vi "TSCAN_CAN_Table.vi"(8 "Data输入":T2={"Communication message"={"Sender"="", "receiver"="", "message"="", "data"=variant}, "Data"={"Config_parameter"={"Bus_Type"=0, "Channel"=0, "Channels used"=0, "DLL_PATH"=path "", "Read message type"=1, "REC_Channel"=0}, "Send_parameter"={"SendData"=[], "Data Length"=0, "ID"=0, "Frame Format"=0, "Frame Type"=0, "BRS"=enum."Close", "FD Frame"=0, "async&sync"=enum."async", "Timeout"=0}, "DBC_Ctr"={"DBC Path"=path "", "DBC loading channel"=0, "DatabaseId"=0, "DBMessages"=[], "DBSignals"=[]}, "CAN_Config_Array"=[], "CANFD_Config_Array"=[], "CAN_Config_Regs_Array"=[], "CANFD_Config_Regs_Array"=[], "Blf_Log"={"Blf_Log_PATH"=path ""}, "UDS"={"UDS Control"={"UDS Channel Index"=0, "Request ID"=1992, "Response ID"=2015, "Request ID (Func)"=1, "Session Mode"=1, "Reset Mode"=255, "DTC Mask"=0, "GropOfDTC"=0, "Seed Level"=2, "Seed"=[], "Key Level"=0, "Key"=[], "Read Identifier"=0, "UDS Read Data"=[], "ASCII Data"="", "Write Identifier"=0, "UDS Wrtie Data"=[], "IO Control Identifier"=1, "UDS IOControl Data"=[], "IO Control Mode"=0, "UDS IOControl Read Data"=[], "Routine Control Identifier"=0, "UDS RoutineControl Data"=[], "UDS RoutineControl Read Data"=[], "Routine Control Mode"=1, "SupportFDCAN"=TRUE, "time config"={"p2_timeout"=0, "p2_extended"=0, "s3_servertime"=0, "s3_clienttime"=0}, "ServiceLayer"={"FilledByte"=0, "STMin"=10, "BlockSize"=10, "FCDelay"=10, "MaxLength"=4095}, "Request"=[], "Respond"=[]}, "DiagModuleIndex"=1984}}, "CAN_Buffer"=[], "CANFD_Buffer"=[], "error in"={"status"=FALSE, "code"=0, "source"=""}, "CAN_Period_Datas"=[], "CANFD_period_Datas"=[], "CAN_Filtering_Datas"=[], "CANFD_Filtering_Datas"=[], "AsynCall?"=FALSE} {"Data"."UDS"."UDS Control"."Respond" format="%.0x"; "Data"."UDS"."UDS Control"."Request" format="%.0x"; "Data"."UDS"."UDS Control"."ServiceLayer"."FilledByte" format="%.0x"; "Data"."UDS"."UDS Control"."GropOfDTC" format="%.0x"; "Data"."UDS"."UDS Control"."DTC Mask" format="%.0x"; "Data"."UDS"."UDS Control"."UDS RoutineControl Read Data" format="%.0x"; "Data"."UDS"."UDS Control"."UDS RoutineControl Data" format="%.0x"; "Data"."UDS"."UDS Control"."Routine Control Identifier" format="%.0x"; "Data"."UDS"."UDS Control"."UDS IOControl Read Data" format="%.0x"; "Data"."UDS"."UDS Control"."UDS IOControl Data" format="%.0x"; "Data"."UDS"."UDS Control"."IO Control Identifier" format="%.0x"; "Data"."UDS"."UDS Control"."UDS Wrtie Data" format="%.0x"; "Data"."UDS"."UDS Control"."UDS Read Data" format="%.0x"; "Data"."UDS"."UDS Control"."Write Identifier" format="%.0x"; "Data"."UDS"."UDS Control"."Read Identifier" format="%.0x"; "Data"."UDS"."UDS Control"."Key" format="%.0x"; "Data"."UDS"."UDS Control"."Seed" format="%.0x"; "Data"."UDS"."UDS Control"."Request ID (Func)" format="%.0x"; "Data"."UDS"."UDS Control"."Response ID" format="%.0x"; "Data"."UDS"."UDS Control"."Request ID" format="%.0x"; "Data"."UDS"."UDS Control"."Session Mode" items=["DefaultSession"=1, "ProgrammingSession"=2, "ExtendedDiagnosticSession"=3]; "Data"."UDS"."UDS Control"."Reset Mode" items=["HardReset"=1, "keyOffOnReset"=2, "SoftReset"=3]; "Data"."UDS"."UDS Control"."IO Control Mode" items=["ReturnControlToECU", "ResetToDefault", "FreezeCurrentState", "ShortTermAdjustment"]; "Data"."UDS"."UDS Control"."Routine Control Mode" items=["Start routine"=1, "Stop routine"=2, "Request routine results"=3]; "Data"."CAN_Config_Regs_Array"."CAN configuration"."AAppChannel" items=["CHN1", "CHN2", "CHN3", "CHN4", "CHN5", "CHN6", "CHN7", "CHN8", "CHN9", "CHN10", "CHN11", "CHN12", "CHN13", "CHN14", "CHN15", "CHN16", "CHN17", "CHN18", "CHN19", "CHN20", "CHN21", "CHN22", "CHN23", "CHN24", "CHN25", "CHN26", "CHN27", "CHN28", "CHN29", "CHN30", "CHN31", "CHN32"]; "Data"."CAN_Config_Regs_Array"."CAN configuration"."AHwChannel" items=["CHN1", "CHN2", "CHN3", "CHN4", "CHN5", "CHN6", "CHN7", "CHN8", "CHN9", "CHN10", "CHN11", "CHN12", "CHN13", "CHN14", "CHN15", "CHN16", "CHN17", "CHN18", "CHN19", "CHN20", "CHN21", "CHN22", "CHN23", "CHN24", "CHN25", "CHN26", "CHN27", "CHN28", "CHN29", "CHN30", "CHN31", "CHN32"]; "Data"."CAN_Config_Regs_Array"."CAN configuration"."HardwareType" items=["BUS_UNKNOWN_TYPE", "TS_TCP_DEVICE", "XL_USB_DEVICE", "TS_USB_DEVICE", "PEAK_USB_DEVICE", "KVASER_USB_DEVICE", "ZLG_USB_DEVICE", "ICS_USB_DEVICE", "TS_TC1005_DEVICE", "CANABLE_USB_DEVICE", "TS_WIRELESS_OBD", "TS_USB_DEVICE_EX", "IXXAT_USB_DEVICE", "TS_ETH_IF_DEVICE", "TS_USB_IF_DEVICE", "BUS_DEV_TYPE_COUNT"]; "Data"."CANFD_Config_Regs_Array"."CANFD Configuration"."Hardware Type" items=["BUS_UNKNOWN_TYPE", "TS_TCP_DEVICE", "XL_USB_DEVICE", "TS_USB_DEVICE", "PEAK_USB_DEVICE", "KVASER_USB_DEVICE", "ZLG_USB_DEVICE", "ICS_USB_DEVICE", "TS_TC1005_DEVICE", "CANABLE_USB_DEVICE", "TS_WIRELESS_OBD", "TS_USB_DEVICE_EX", "IXXAT_USB_DEVICE", "TS_ETH_IF_DEVICE", "TS_USB_IF_DEVICE", "BUS_DEV_TYPE_COUNT"]; "Data"."CANFD_Config_Regs_Array"."CANFD Configuration"."AHwChannel" items=["CHN1", "CHN2", "CHN3", "CHN4", "CHN5", "CHN6", "CHN7", "CHN8", "CHN9", "CHN10", "CHN11", "CHN12", "CHN13", "CHN14", "CHN15", "CHN16", "CHN17", "CHN18", "CHN19", "CHN20", "CHN21", "CHN22", "CHN23", "CHN24", "CHN25", "CHN26", "CHN27", "CHN28", "CHN29", "CHN30", "CHN31", "CHN32"]; "Data"."CANFD_Config_Regs_Array"."CANFD Configuration"."AAppChannel" items=["CHN1", "CHN2", "CHN3", "CHN4", "CHN5", "CHN6", "CHN7", "CHN8", "CHN9", "CHN10", "CHN11", "CHN12", "CHN13", "CHN14", "CHN15", "CHN16", "CHN17", "CHN18", "CHN19", "CHN20", "CHN21", "CHN22", "CHN23", "CHN24", "CHN25", "CHN26", "CHN27", "CHN28", "CHN29", "CHN30", "CHN31", "CHN32"]; "Data"."CANFD_Config_Regs_Array"."CANFD Configuration"."AControllerType" items=["lfdtCAN", "lfdtISOFDCAN", "lfdtNonISOFDFDCAN"]; "Data"."CANFD_Config_Regs_Array"."CANFD Configuration"."AControllerMode" items=["lfdmNormal", "lfdmACKOff", "lfdmRestricted"]; "Data"."CANFD_Config_Array"."Hardware Type" items=["BUS_UNKNOWN_TYPE", "TS_TCP_DEVICE", "XL_USB_DEVICE", "TS_USB_DEVICE", "PEAK_USB_DEVICE", "KVASER_USB_DEVICE", "ZLG_USB_DEVICE", "ICS_USB_DEVICE", "TS_TC1005_DEVICE", "CANABLE_USB_DEVICE", "TS_WIRELESS_OBD", "TS_USB_DEVICE_EX", "IXXAT_USB_DEVICE", "TS_ETH_IF_DEVICE", "TS_USB_IF_DEVICE", "BUS_DEV_TYPE_COUNT"]; "Data"."CANFD_Config_Array"."AHwChannel" items=["CHN1", "CHN2", "CHN3", "CHN4", "CHN5", "CHN6", "CHN7", "CHN8", "CHN9", "CHN10", "CHN11", "CHN12", "CHN13", "CHN14", "CHN15", "CHN16", "CHN17", "CHN18", "CHN19", "CHN20", "CHN21", "CHN22", "CHN23", "CHN24", "CHN25", "CHN26", "CHN27", "CHN28", "CHN29", "CHN30", "CHN31", "CHN32"]; "Data"."CANFD_Config_Array"."AAppChannel" items=["CHN1", "CHN2", "CHN3", "CHN4", "CHN5", "CHN6", "CHN7", "CHN8", "CHN9", "CHN10", "CHN11", "CHN12", "CHN13", "CHN14", "CHN15", "CHN16", "CHN17", "CHN18", "CHN19", "CHN20", "CHN21", "CHN22", "CHN23", "CHN24", "CHN25", "CHN26", "CHN27", "CHN28", "CHN29", "CHN30", "CHN31", "CHN32"]; "Data"."CANFD_Config_Array"."AControllerType" items=["lfdtCAN", "lfdtISOFDCAN", "lfdtNonISOFDFDCAN"]; "Data"."CANFD_Config_Array"."AControllerMode" items=["lfdmNormal", "lfdmACKOff", "lfdmRestricted"]; "Data"."CAN_Config_Array"."AAppChannel" items=["CHN1", "CHN2", "CHN3", "CHN4", "CHN5", "CHN6", "CHN7", "CHN8", "CHN9", "CHN10", "CHN11", "CHN12", "CHN13", "CHN14", "CHN15", "CHN16", "CHN17", "CHN18", "CHN19", "CHN20", "CHN21", "CHN22", "CHN23", "CHN24", "CHN25", "CHN26", "CHN27", "CHN28", "CHN29", "CHN30", "CHN31", "CHN32"]; "Data"."CAN_Config_Array"."AHwChannel" items=["CHN1", "CHN2", "CHN3", "CHN4", "CHN5", "CHN6", "CHN7", "CHN8", "CHN9", "CHN10", "CHN11", "CHN12", "CHN13", "CHN14", "CHN15", "CHN16", "CHN17", "CHN18", "CHN19", "CHN20", "CHN21", "CHN22", "CHN23", "CHN24", "CHN25", "CHN26", "CHN27", "CHN28", "CHN29", "CHN30", "CHN31", "CHN32"]; "Data"."CAN_Config_Array"."HardwareType" items=["BUS_UNKNOWN_TYPE", "TS_TCP_DEVICE", "XL_USB_DEVICE", "TS_USB_DEVICE", "PEAK_USB_DEVICE", "KVASER_USB_DEVICE", "ZLG_USB_DEVICE", "ICS_USB_DEVICE", "TS_TC1005_DEVICE", "CANABLE_USB_DEVICE", "TS_WIRELESS_OBD", "TS_USB_DEVICE_EX", "IXXAT_USB_DEVICE", "TS_ETH_IF_DEVICE", "TS_USB_IF_DEVICE", "BUS_DEV_TYPE_COUNT"]; "Data"."DBC_Ctr"."DBSignals"."SignalList"."Message_Type" items=["CAN", "CANFD", "J1939"]; "Data"."DBC_Ctr"."DBSignals"."SignalList"."Mux_Type" items=["Normal", "multiplexor", "multiplexed"]; "Data"."DBC_Ctr"."DBSignals"."SignalList"."Is_Motorola" items=["Intel", "Motorola"]; "Data"."DBC_Ctr"."DBSignals"."SignalList"."Value_Type" items=["unsigned int", "signed int", "float", "double"]; "Data"."DBC_Ctr"."DBSignals"."SignalList"."ID" format="%.0x"; "Data"."DBC_Ctr"."DBMessages"."BRS" items=["No BRS", "BRS"]; "Data"."DBC_Ctr"."DBMessages"."ID" format="%.0x"; "Data"."DBC_Ctr"."DBMessages"."Type" items=["cftStdCAN", "cftExtCAN", "cftJ1939", "cftStdCANFD", "cftExtCANFD"]; "Data"."DBC_Ctr"."DBC loading channel" items=["CHN1", "CHN2", "CHN3", "CHN4", "CHN5", "CHN6", "CHN7", "CHN8", "CHN9", "CHN10", "CHN11", "CHN12", "CHN13", "CHN14", "CHN15", "CHN16", "CHN17", "CHN18", "CHN19", "CHN20", "CHN21", "CHN22", "CHN23", "CHN24", "CHN25", "CHN26", "CHN27", "CHN28", "CHN29", "CHN30", "CHN31", "CHN32"]; "Data"."Send_parameter"."FD Frame" items=["Ordinary CAN Data", "FD CAN Data"]; "Data"."Send_parameter"."Frame Type" items=["Standard Frame", "Extended Frame"]; "Data"."Send_parameter"."Frame Format" items=["Standard Frame", "Extended Frame"]; "Data"."Send_parameter"."ID" format="%x"; "Data"."Send_parameter"."Data Length" items=["0", "1", "2", "3", "4", "5", "6", "7", "8", "12", "16", "20", "24", "32", "48", "64"]; "Data"."Send_parameter"."SendData" format="%x"; "Data"."Config_parameter"."REC_Channel" items=["CHN1", "CHN2", "CHN3", "CHN4", "CHN5", "CHN6", "CHN7", "CHN8", "CHN9", "CHN10", "CHN11", "CHN12", "CHN13", "CHN14", "CHN15", "CHN16", "CHN17", "CHN18", "CHN19", "CHN20", "CHN21", "CHN22", "CHN23", "CHN24", "CHN25", "CHN26", "CHN27", "CHN28", "CHN29", "CHN30", "CHN31", "CHN32"]; "Data"."Config_parameter"."Read message type" items=["Only read received messages", "Receive&send messages"]; "Data"."Config_parameter"."Channels used" items=["1 Channel"=1, "2 Channels"=2, "3 Channels"=3, "4 Channels"=4, "5 Channels"=5, "6 Channels"=6, "7 Channels"=7, "8 Channels"=8, "9 Channels"=9, "10 Channels"=10, "11 Channels"=11, "12 Channels"=12, "13 Channels"=13, "14 Channels"=14, "15 Channels"=15, "16 Channels"=16]; "Data"."Config_parameter"."Channel" items=["Disable", "Enable"]; "Data"."Config_parameter"."Bus_Type" items=["CAN", "CANFD"]}, 9 "Fold Data":bool, 10 "ACANMsgBuffer":T1(array[cluster]), 11 "MCListbox reference handle":refnum<vi>) -> (0 "Data输出":T2={"Communication message"={"Sender"="", "receiver"="", "message"="", "data"=variant}, "Data"={"Config_parameter"={"Bus_Type"=0, "Channel"=0, "Channels used"=0, "DLL_PATH"=path "", "Read message type"=1, "REC_Channel"=0}, "Send_parameter"={"SendData"=[], "Data Length"=0, "ID"=0, "Frame Format"=0, "Frame Type"=0, "BRS"=enum."Close", "FD Frame"=0, "async&sync"=enum."async", "Timeout"=0}, "DBC_Ctr"={"DBC Path"=path "", "DBC loading channel"=0, "DatabaseId"=0, "DBMessages"=[], "DBSignals"=[]}, "CAN_Config_Array"=[], "CANFD_Config_Array"=[], "CAN_Config_Regs_Array"=[], "CANFD_Config_Regs_Array"=[], "Blf_Log"={"Blf_Log_PATH"=path ""}, "UDS"={"UDS Control"={"UDS Channel Index"=0, "Request ID"=1992, "Response ID"=2015, "Request ID (Func)"=1, "Session Mode"=1, "Reset Mode"=255, "DTC Mask"=0, "GropOfDTC"=0, "Seed Level"=2, "Seed"=[], "Key Level"=0, "Key"=[], "Read Identifier"=0, "UDS Read Data"=[], "ASCII Data"="", "Write Identifier"=0, "UDS Wrtie Data"=[], "IO Control Identifier"=1, "UDS IOControl Data"=[], "IO Control Mode"=0, "UDS IOControl Read Data"=[], "Routine Control Identifier"=0, "UDS RoutineControl Data"=[], "UDS RoutineControl Read Data"=[], "Routine Control Mode"=1, "SupportFDCAN"=TRUE, "time config"={"p2_timeout"=0, "p2_extended"=0, "s3_servertime"=0, "s3_clienttime"=0}, "ServiceLayer"={"FilledByte"=0, "STMin"=10, "BlockSize"=10, "FCDelay"=10, "MaxLength"=4095}, "Request"=[], "Respond"=[]}, "DiagModuleIndex"=1984}}, "CAN_Buffer"=[], "CANFD_Buffer"=[], "error in"={"status"=FALSE, "code"=0, "source"=""}, "CAN_Period_Datas"=[], "CANFD_period_Datas"=[], "CAN_Filtering_Datas"=[], "CANFD_Filtering_Datas"=[], "AsynCall?"=FALSE} {"Data"."UDS"."UDS Control"."Respond" format="%.0x"; "Data"."UDS"."UDS Control"."Request" format="%.0x"; "Data"."UDS"."UDS Control"."ServiceLayer"."FilledByte" format="%.0x"; "Data"."UDS"."UDS Control"."GropOfDTC" format="%.0x"; "Data"."UDS"."UDS Control"."DTC Mask" format="%.0x"; "Data"."UDS"."UDS Control"."UDS RoutineControl Read Data" format="%.0x"; "Data"."UDS"."UDS Control"."UDS RoutineControl Data" format="%.0x"; "Data"."UDS"."UDS Control"."Routine Control Identifier" format="%.0x"; "Data"."UDS"."UDS Control"."UDS IOControl Read Data" format="%.0x"; "Data"."UDS"."UDS Control"."UDS IOControl Data" format="%.0x"; "Data"."UDS"."UDS Control"."IO Control Identifier" format="%.0x"; "Data"."UDS"."UDS Control"."UDS Wrtie Data" format="%.0x"; "Data"."UDS"."UDS Control"."UDS Read Data" format="%.0x"; "Data"."UDS"."UDS Control"."Write Identifier" format="%.0x"; "Data"."UDS"."UDS Control"."Read Identifier" format="%.0x"; "Data"."UDS"."UDS Control"."Key" format="%.0x"; "Data"."UDS"."UDS Control"."Seed" format="%.0x"; "Data"."UDS"."UDS Control"."Request ID (Func)" format="%.0x"; "Data"."UDS"."UDS Control"."Response ID" format="%.0x"; "Data"."UDS"."UDS Control"."Request ID" format="%.0x"; "Data"."UDS"."UDS Control"."Session Mode" items=["DefaultSession"=1, "ProgrammingSession"=2, "ExtendedDiagnosticSession"=3]; "Data"."UDS"."UDS Control"."Reset Mode" items=["HardReset"=1, "keyOffOnReset"=2, "SoftReset"=3]; "Data"."UDS"."UDS Control"."IO Control Mode" items=["ReturnControlToECU", "ResetToDefault", "FreezeCurrentState", "ShortTermAdjustment"]; "Data"."UDS"."UDS Control"."Routine Control Mode" items=["Start routine"=1, "Stop routine"=2, "Request routine results"=3]; "Data"."CAN_Config_Regs_Array"."CAN configuration"."AAppChannel" items=["CHN1", "CHN2", "CHN3", "CHN4", "CHN5", "CHN6", "CHN7", "CHN8", "CHN9", "CHN10", "CHN11", "CHN12", "CHN13", "CHN14", "CHN15", "CHN16", "CHN17", "CHN18", "CHN19", "CHN20", "CHN21", "CHN22", "CHN23", "CHN24", "CHN25", "CHN26", "CHN27", "CHN28", "CHN29", "CHN30", "CHN31", "CHN32"]; "Data"."CAN_Config_Regs_Array"."CAN configuration"."AHwChannel" items=["CHN1", "CHN2", "CHN3", "CHN4", "CHN5", "CHN6", "CHN7", "CHN8", "CHN9", "CHN10", "CHN11", "CHN12", "CHN13", "CHN14", "CHN15", "CHN16", "CHN17", "CHN18", "CHN19", "CHN20", "CHN21", "CHN22", "CHN23", "CHN24", "CHN25", "CHN26", "CHN27", "CHN28", "CHN29", "CHN30", "CHN31", "CHN32"]; "Data"."CAN_Config_Regs_Array"."CAN configuration"."HardwareType" items=["BUS_UNKNOWN_TYPE", "TS_TCP_DEVICE", "XL_USB_DEVICE", "TS_USB_DEVICE", "PEAK_USB_DEVICE", "KVASER_USB_DEVICE", "ZLG_USB_DEVICE", "ICS_USB_DEVICE", "TS_TC1005_DEVICE", "CANABLE_USB_DEVICE", "TS_WIRELESS_OBD", "TS_USB_DEVICE_EX", "IXXAT_USB_DEVICE", "TS_ETH_IF_DEVICE", "TS_USB_IF_DEVICE", "BUS_DEV_TYPE_COUNT"]; "Data"."CANFD_Config_Regs_Array"."CANFD Configuration"."Hardware Type" items=["BUS_UNKNOWN_TYPE", "TS_TCP_DEVICE", "XL_USB_DEVICE", "TS_USB_DEVICE", "PEAK_USB_DEVICE", "KVASER_USB_DEVICE", "ZLG_USB_DEVICE", "ICS_USB_DEVICE", "TS_TC1005_DEVICE", "CANABLE_USB_DEVICE", "TS_WIRELESS_OBD", "TS_USB_DEVICE_EX", "IXXAT_USB_DEVICE", "TS_ETH_IF_DEVICE", "TS_USB_IF_DEVICE", "BUS_DEV_TYPE_COUNT"]; "Data"."CANFD_Config_Regs_Array"."CANFD Configuration"."AHwChannel" items=["CHN1", "CHN2", "CHN3", "CHN4", "CHN5", "CHN6", "CHN7", "CHN8", "CHN9", "CHN10", "CHN11", "CHN12", "CHN13", "CHN14", "CHN15", "CHN16", "CHN17", "CHN18", "CHN19", "CHN20", "CHN21", "CHN22", "CHN23", "CHN24", "CHN25", "CHN26", "CHN27", "CHN28", "CHN29", "CHN30", "CHN31", "CHN32"]; "Data"."CANFD_Config_Regs_Array"."CANFD Configuration"."AAppChannel" items=["CHN1", "CHN2", "CHN3", "CHN4", "CHN5", "CHN6", "CHN7", "CHN8", "CHN9", "CHN10", "CHN11", "CHN12", "CHN13", "CHN14", "CHN15", "CHN16", "CHN17", "CHN18", "CHN19", "CHN20", "CHN21", "CHN22", "CHN23", "CHN24", "CHN25", "CHN26", "CHN27", "CHN28", "CHN29", "CHN30", "CHN31", "CHN32"]; "Data"."CANFD_Config_Regs_Array"."CANFD Configuration"."AControllerType" items=["lfdtCAN", "lfdtISOFDCAN", "lfdtNonISOFDFDCAN"]; "Data"."CANFD_Config_Regs_Array"."CANFD Configuration"."AControllerMode" items=["lfdmNormal", "lfdmACKOff", "lfdmRestricted"]; "Data"."CANFD_Config_Array"."Hardware Type" items=["BUS_UNKNOWN_TYPE", "TS_TCP_DEVICE", "XL_USB_DEVICE", "TS_USB_DEVICE", "PEAK_USB_DEVICE", "KVASER_USB_DEVICE", "ZLG_USB_DEVICE", "ICS_USB_DEVICE", "TS_TC1005_DEVICE", "CANABLE_USB_DEVICE", "TS_WIRELESS_OBD", "TS_USB_DEVICE_EX", "IXXAT_USB_DEVICE", "TS_ETH_IF_DEVICE", "TS_USB_IF_DEVICE", "BUS_DEV_TYPE_COUNT"]; "Data"."CANFD_Config_Array"."AHwChannel" items=["CHN1", "CHN2", "CHN3", "CHN4", "CHN5", "CHN6", "CHN7", "CHN8", "CHN9", "CHN10", "CHN11", "CHN12", "CHN13", "CHN14", "CHN15", "CHN16", "CHN17", "CHN18", "CHN19", "CHN20", "CHN21", "CHN22", "CHN23", "CHN24", "CHN25", "CHN26", "CHN27", "CHN28", "CHN29", "CHN30", "CHN31", "CHN32"]; "Data"."CANFD_Config_Array"."AAppChannel" items=["CHN1", "CHN2", "CHN3", "CHN4", "CHN5", "CHN6", "CHN7", "CHN8", "CHN9", "CHN10", "CHN11", "CHN12", "CHN13", "CHN14", "CHN15", "CHN16", "CHN17", "CHN18", "CHN19", "CHN20", "CHN21", "CHN22", "CHN23", "CHN24", "CHN25", "CHN26", "CHN27", "CHN28", "CHN29", "CHN30", "CHN31", "CHN32"]; "Data"."CANFD_Config_Array"."AControllerType" items=["lfdtCAN", "lfdtISOFDCAN", "lfdtNonISOFDFDCAN"]; "Data"."CANFD_Config_Array"."AControllerMode" items=["lfdmNormal", "lfdmACKOff", "lfdmRestricted"]; "Data"."CAN_Config_Array"."AAppChannel" items=["CHN1", "CHN2", "CHN3", "CHN4", "CHN5", "CHN6", "CHN7", "CHN8", "CHN9", "CHN10", "CHN11", "CHN12", "CHN13", "CHN14", "CHN15", "CHN16", "CHN17", "CHN18", "CHN19", "CHN20", "CHN21", "CHN22", "CHN23", "CHN24", "CHN25", "CHN26", "CHN27", "CHN28", "CHN29", "CHN30", "CHN31", "CHN32"]; "Data"."CAN_Config_Array"."AHwChannel" items=["CHN1", "CHN2", "CHN3", "CHN4", "CHN5", "CHN6", "CHN7", "CHN8", "CHN9", "CHN10", "CHN11", "CHN12", "CHN13", "CHN14", "CHN15", "CHN16", "CHN17", "CHN18", "CHN19", "CHN20", "CHN21", "CHN22", "CHN23", "CHN24", "CHN25", "CHN26", "CHN27", "CHN28", "CHN29", "CHN30", "CHN31", "CHN32"]; "Data"."CAN_Config_Array"."HardwareType" items=["BUS_UNKNOWN_TYPE", "TS_TCP_DEVICE", "XL_USB_DEVICE", "TS_USB_DEVICE", "PEAK_USB_DEVICE", "KVASER_USB_DEVICE", "ZLG_USB_DEVICE", "ICS_USB_DEVICE", "TS_TC1005_DEVICE", "CANABLE_USB_DEVICE", "TS_WIRELESS_OBD", "TS_USB_DEVICE_EX", "IXXAT_USB_DEVICE", "TS_ETH_IF_DEVICE", "TS_USB_IF_DEVICE", "BUS_DEV_TYPE_COUNT"]; "Data"."DBC_Ctr"."DBSignals"."SignalList"."Message_Type" items=["CAN", "CANFD", "J1939"]; "Data"."DBC_Ctr"."DBSignals"."SignalList"."Mux_Type" items=["Normal", "multiplexor", "multiplexed"]; "Data"."DBC_Ctr"."DBSignals"."SignalList"."Is_Motorola" items=["Intel", "Motorola"]; "Data"."DBC_Ctr"."DBSignals"."SignalList"."Value_Type" items=["unsigned int", "signed int", "float", "double"]; "Data"."DBC_Ctr"."DBSignals"."SignalList"."ID" format="%.0x"; "Data"."DBC_Ctr"."DBMessages"."BRS" items=["No BRS", "BRS"]; "Data"."DBC_Ctr"."DBMessages"."ID" format="%.0x"; "Data"."DBC_Ctr"."DBMessages"."Type" items=["cftStdCAN", "cftExtCAN", "cftJ1939", "cftStdCANFD", "cftExtCANFD"]; "Data"."DBC_Ctr"."DBC loading channel" items=["CHN1", "CHN2", "CHN3", "CHN4", "CHN5", "CHN6", "CHN7", "CHN8", "CHN9", "CHN10", "CHN11", "CHN12", "CHN13", "CHN14", "CHN15", "CHN16", "CHN17", "CHN18", "CHN19", "CHN20", "CHN21", "CHN22", "CHN23", "CHN24", "CHN25", "CHN26", "CHN27", "CHN28", "CHN29", "CHN30", "CHN31", "CHN32"]; "Data"."Send_parameter"."FD Frame" items=["Ordinary CAN Data", "FD CAN Data"]; "Data"."Send_parameter"."Frame Type" items=["Standard Frame", "Extended Frame"]; "Data"."Send_parameter"."Frame Format" items=["Standard Frame", "Extended Frame"]; "Data"."Send_parameter"."ID" format="%x"; "Data"."Send_parameter"."Data Length" items=["0", "1", "2", "3", "4", "5", "6", "7", "8", "12", "16", "20", "24", "32", "48", "64"]; "Data"."Send_parameter"."SendData" format="%x"; "Data"."Config_parameter"."REC_Channel" items=["CHN1", "CHN2", "CHN3", "CHN4", "CHN5", "CHN6", "CHN7", "CHN8", "CHN9", "CHN10", "CHN11", "CHN12", "CHN13", "CHN14", "CHN15", "CHN16", "CHN17", "CHN18", "CHN19", "CHN20", "CHN21", "CHN22", "CHN23", "CHN24", "CHN25", "CHN26", "CHN27", "CHN28", "CHN29", "CHN30", "CHN31", "CHN32"]; "Data"."Config_parameter"."Read message type" items=["Only read received messages", "Receive&send messages"]; "Data"."Config_parameter"."Channels used" items=["1 Channel"=1, "2 Channels"=2, "3 Channels"=3, "4 Channels"=4, "5 Channels"=5, "6 Channels"=6, "7 Channels"=7, "8 Channels"=8, "9 Channels"=9, "10 Channels"=10, "11 Channels"=11, "12 Channels"=12, "13 Channels"=13, "14 Channels"=14, "15 Channels"=15, "16 Channels"=16]; "Data"."Config_parameter"."Channel" items=["Disable", "Enable"]; "Data"."Config_parameter"."Bus_Type" items=["CAN", "CANFD"]})   [LabVIEW 2014]
uses:
  Utilities/Typedef/Hardware_Subtype.ctl
  Typedef/TSCAN_Config_parameter.ctl
  Typedef/TSCAN_Send_parameter.ctl
  Typedef/TSCAN_CAN_CANFD_Demo_Data.ctl
  Typedef/TSCAN_CAN_CANFD_Demo_Data1.ctl
  Typedef/TSCAN_DBC_Ctr.ctl
  Typedef/TSCAN_CAN_Configuration.ctl
  Typedef/TSCAN_CANFD_Configuration.ctl
  Typedef/TSCAN_CANFD_Configuration_Regs.ctl
  Typedef/TSCAN_CAN_Configuration_Regs.ctl
  All_Control/Typedef/Hardware Type.ctl
  All_Control/Typedef/Blf_Log.ctl
  DataBase/Typedef/DBMessage.ctl
  DataBase/Typedef/DBSignal.ctl
  Diagnosis/Typedef/UDS Control.ctl
  Diagnosis/Typedef/UDS Cluster.ctl
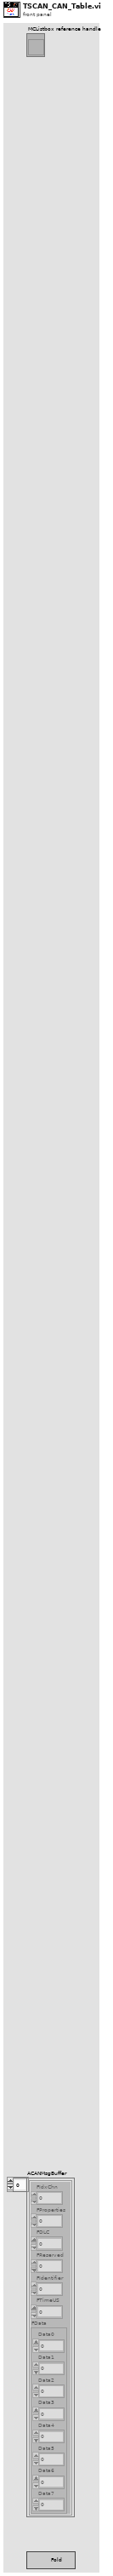
[diagram p1: front panel]
types:
  T1 = cluster{"FIdxChn":u8, "FProperties":u8, "FDLC":u8, "FReserved":u8, "FIdentifier":i32, "FTimeUS":u64, "FData":cluster{"Data0":u8, "Data1":u8, "Data2":u8, "Data3":u8, "Data4":u8, "Data5":u8, "Data6":u8, "Data7":u8}}[]
  T2 = typedef "TSCAN_CAN_CANFD_Demo_Data1.ctl" = cluster{"Communication message":cluster{"Sender":string, "receiver":string, "message":string, "data":variant}, "Data":T3, "CAN_Buffer":cluster{"FIdxChn":u8, "FProperties":u8, "FDLC":u8, "FReserved":u8, "FIdentifier":i32, "FTimeUS":u64, "FData":cluster{"Data0":u8, "Data1":u8, "Data2":u8, "Data3":u8, "Data4":u8, "Data5":u8, "Data6":u8, "Data7":u8}}[], "CANFD_Buffer":cluster{"FIdxChn":u8, "FProperties":u8, "FDLC":u8, "FReserved":u8, "FIdentifier":i32, "FTimeUS":u64, "FDatas":cluster{"Initialize array[0]":u8, "Initialize array[1]":u8, "Initialize array[2]":u8, "Initialize array[3]":u8, "Initialize array[4]":u8, "Initialize array[5]":u8, "Initialize array[6]":u8, "Initialize array[7]":u8, "Initialize array[8]":u8, "Initialize array[9]":u8, "Initialize array[10]":u8, "Initialize array[11]":u8, "Initialize array[12]":u8, "Initialize array[13]":u8, "Initialize array[14]":u8, "Initialize array[15]":u8, "Initialize array[16]":u8, "Initialize array[17]":u8, "Initialize array[18]":u8, "Initialize array[19]":u8, "Initialize array[20]":u8, "Initialize array[21]":u8, "Initialize array[22]":u8, "Initialize array[23]":u8, "Initialize array[24]":u8, "Initialize array[25]":u8, "Initialize array[26]":u8, "Initialize array[27]":u8, "Initialize array[28]":u8, "Initialize array[29]":u8, "Initialize array[30]":u8, "Initialize array[31]":u8, "Initialize array[32]":u8, "Initialize array[33]":u8, "Initialize array[34]":u8, "Initialize array[35]":u8, "Initialize array[36]":u8, "Initialize array[37]":u8, "Initialize array[38]":u8, "Initialize array[39]":u8, "Initialize array[40]":u8, "Initialize array[41]":u8, "Initialize array[42]":u8, "Initialize array[43]":u8, "Initialize array[44]":u8, "Initialize array[45]":u8, "Initialize array[46]":u8, "Initialize array[47]":u8, "Initialize array[48]":u8, "Initialize array[49]":u8, "Initialize array[50]":u8, "Initialize array[51]":u8, "Initialize array[52]":u8, "Initialize array[53]":u8, "Initialize array[54]":u8, "Initialize array[55]":u8, "Initialize array[56]":u8, "Initialize array[57]":u8, "Initialize array[58]":u8, "Initialize array[59]":u8, "Initialize array[60]":u8, "Initialize array[61]":u8, "Initialize array[62]":u8, "Initialize array[63]":u8}}[], "error in":errorcluster, "CAN_Period_Datas":cluster{"FIdxChn":u8, "FProperties":u8, "FDLC":u8, "FReserved":u8, "FIdentifier":i32, "FTimeUS":u64, "FData":cluster{"Data0":u8, "Data1":u8, "Data2":u8, "Data3":u8, "Data4":u8, "Data5":u8, "Data6":u8, "Data7":u8}}[], "CANFD_period_Datas":cluster{"FIdxChn":u8, "FProperties":u8, "FDLC":u8, "FReserved":u8, "FIdentifier":i32, "FTimeUS":u64, "FDatas":cluster{"Initialize array[0]":u8, "Initialize array[1]":u8, "Initialize array[2]":u8, "Initialize array[3]":u8, "Initialize array[4]":u8, "Initialize array[5]":u8, "Initialize array[6]":u8, "Initialize array[7]":u8, "Initialize array[8]":u8, "Initialize array[9]":u8, "Initialize array[10]":u8, "Initialize array[11]":u8, "Initialize array[12]":u8, "Initialize array[13]":u8, "Initialize array[14]":u8, "Initialize array[15]":u8, "Initialize array[16]":u8, "Initialize array[17]":u8, "Initialize array[18]":u8, "Initialize array[19]":u8, "Initialize array[20]":u8, "Initialize array[21]":u8, "Initialize array[22]":u8, "Initialize array[23]":u8, "Initialize array[24]":u8, "Initialize array[25]":u8, "Initialize array[26]":u8, "Initialize array[27]":u8, "Initialize array[28]":u8, "Initialize array[29]":u8, "Initialize array[30]":u8, "Initialize array[31]":u8, "Initialize array[32]":u8, "Initialize array[33]":u8, "Initialize array[34]":u8, "Initialize array[35]":u8, "Initialize array[36]":u8, "Initialize array[37]":u8, "Initialize array[38]":u8, "Initialize array[39]":u8, "Initialize array[40]":u8, "Initialize array[41]":u8, "Initialize array[42]":u8, "Initialize array[43]":u8, "Initialize array[44]":u8, "Initialize array[45]":u8, "Initialize array[46]":u8, "Initialize array[47]":u8, "Initialize array[48]":u8, "Initialize array[49]":u8, "Initialize array[50]":u8, "Initialize array[51]":u8, "Initialize array[52]":u8, "Initialize array[53]":u8, "Initialize array[54]":u8, "Initialize array[55]":u8, "Initialize array[56]":u8, "Initialize array[57]":u8, "Initialize array[58]":u8, "Initialize array[59]":u8, "Initialize array[60]":u8, "Initialize array[61]":u8, "Initialize array[62]":u8, "Initialize array[63]":u8}}[], "CAN_Filtering_Datas":cluster{"FIdxChn":u8, "FProperties":u8, "FDLC":u8, "FReserved":u8, "FIdentifier":i32, "FTimeUS":u64, "FData":cluster{"Data0":u8, "Data1":u8, "Data2":u8, "Data3":u8, "Data4":u8, "Data5":u8, "Data6":u8, "Data7":u8}}[], "CANFD_Filtering_Datas":cluster{"FIdxChn":u8, "FProperties":u8, "FDLC":u8, "FReserved":u8, "FIdentifier":i32, "FTimeUS":u64, "FDatas":cluster{"Initialize array[0]":u8, "Initialize array[1]":u8, "Initialize array[2]":u8, "Initialize array[3]":u8, "Initialize array[4]":u8, "Initialize array[5]":u8, "Initialize array[6]":u8, "Initialize array[7]":u8, "Initialize array[8]":u8, "Initialize array[9]":u8, "Initialize array[10]":u8, "Initialize array[11]":u8, "Initialize array[12]":u8, "Initialize array[13]":u8, "Initialize array[14]":u8, "Initialize array[15]":u8, "Initialize array[16]":u8, "Initialize array[17]":u8, "Initialize array[18]":u8, "Initialize array[19]":u8, "Initialize array[20]":u8, "Initialize array[21]":u8, "Initialize array[22]":u8, "Initialize array[23]":u8, "Initialize array[24]":u8, "Initialize array[25]":u8, "Initialize array[26]":u8, "Initialize array[27]":u8, "Initialize array[28]":u8, "Initialize array[29]":u8, "Initialize array[30]":u8, "Initialize array[31]":u8, "Initialize array[32]":u8, "Initialize array[33]":u8, "Initialize array[34]":u8, "Initialize array[35]":u8, "Initialize array[36]":u8, "Initialize array[37]":u8, "Initialize array[38]":u8, "Initialize array[39]":u8, "Initialize array[40]":u8, "Initialize array[41]":u8, "Initialize array[42]":u8, "Initialize array[43]":u8, "Initialize array[44]":u8, "Initialize array[45]":u8, "Initialize array[46]":u8, "Initialize array[47]":u8, "Initialize array[48]":u8, "Initialize array[49]":u8, "Initialize array[50]":u8, "Initialize array[51]":u8, "Initialize array[52]":u8, "Initialize array[53]":u8, "Initialize array[54]":u8, "Initialize array[55]":u8, "Initialize array[56]":u8, "Initialize array[57]":u8, "Initialize array[58]":u8, "Initialize array[59]":u8, "Initialize array[60]":u8, "Initialize array[61]":u8, "Initialize array[62]":u8, "Initialize array[63]":u8}}[], "AsynCall?":bool}
  T3 = typedef "TSCAN_CAN_CANFD_Demo_Data.ctl" = cluster{"Config_parameter":T4, "Send_parameter":T5, "DBC_Ctr":T6, "CAN_Config_Array":T9[], "CANFD_Config_Array":T12[], "CAN_Config_Regs_Array":T13[], "CANFD_Config_Regs_Array":T14[], "Blf_Log":T15, "UDS":T16}
  T4 = typedef "TSCAN_Config_parameter.ctl" = cluster{"Bus_Type":u16, "Channel":i32, "Channels used":u16, "DLL_PATH":path, "Read message type":u16, "REC_Channel":i32}
  T5 = typedef "TSCAN_Send_parameter.ctl" = cluster{"SendData":u8[], "Data Length":i32, "ID":i32, "Frame Format":u8, "Frame Type":u8, "BRS":enum16{"Close", "Open"}, "FD Frame":u8, "async&sync":enum16{"async", "sync"}, "Timeout":u16}
  T6 = typedef "TSCAN_DBC_Ctr.ctl" = cluster{"DBC Path":path, "DBC loading channel":i32, "DatabaseId":u32, "DBMessages":T7[], "DBSignals":cluster{"MessageName":string, "SignalList":T8[]}[]}
  T7 = typedef "DBMessage.ctl" = cluster{"Type":u16, "DLC":i32, "ID":i32, "CycleTime":dbl, "Name":string, "Comment":string, "TX_Node_Index":i32, "Owned_Signal_List_Count ":i32, "Owned_Signal_List_Signal_Index":i32, "BRS":i32}
  T8 = typedef "DBSignal.ctl" = cluster{"ID":i32, "Value_Type":i32, "Is_Motorola":i32, "ValTab_Index":i32, "Mux_Type":i32, "Mux_Value":dbl, "Layout_Start":i32, "Length":i32, "Factor":dbl, "Offset":dbl, "InitValue":dbl, "Min":dbl, "Max":dbl, "Name":string, "Unit":string, "Comment":string, "Message_Index":i32, "Message_Type":i32}
  T9 = typedef "TSCAN_CAN_Configuration.ctl" = cluster{"HardwareType":T10, "Hardware Subtype":T11, "ABaudrateKbps":sgl, "AListenOnly":enum16{"Normal", "ListenOnly"}, "Int120Ohm":enum16{"Disable", "Enable"}, "EnableChannel":enum16{"Disable", "Enable"}, "AHwChannel":i32, "AAppChannel":i32, "AldHW":i32}
  T10 = typedef "Hardware Type.ctl" = i32
  T11 = typedef "Hardware_Subtype.ctl" = enum16{"TS_UNKNOWN_DEVICE", "TSCAN_PRO", "TSCAN_Lite1", "TC1001", "TL1001", "TC1011", "TM5011", "TC1002", "TC1014", "TSCANFD2517", "TC1026", "TC1016", "TC1012", "TC1013", "TLog1002", "TC1034", "TC1018", "GW2116", "TC2115", "MP1013", "TC1113", "TC1114", "TP1013", "TC1017", "TP1018", "TF10XX", "TL1004_FD_4_LIN_2", "TE1051", "TP1051", "TP1034", "TTS9015", "TP1026", "TTS1026", "TTS1034", "TTS1018", "TL1011", "TTS1015_LiAuto", "TTS1013_LiAuto", "TTS1016Pro", "TC1054Pro", "TC1054", "TLog1038", "TO1013", "TC1034Pro", "TC1018Pro", "TC1038Pro", "TS_DEV_END"}
  T12 = typedef "TSCAN_CANFD_Configuration.ctl" = cluster{"Hardware Type":T10, "Hardware Subtype":T11, "AArbRateKbps":sgl, "AListenOnly":enum16{"Normal", "ListenOnly"}, "Int120Ohm":enum16{"Disable", "Enable"}, "EnableChannel":enum16{"Disable", "Enable"}, "AHwChannel":i32, "AAppChannel":i32, "ADataRateKbps":sgl, "AControllerType":i32, "AControllerMode":i32, "AldHW":i32}
  T13 = typedef "TSCAN_CAN_Configuration_Regs.ctl" = cluster{"CAN_Sampling point":cluster{"ASEG1":i32, "ASEG2":i32, "APrescaler":i32, "ASJW":i32}, "CAN configuration":T9}
  T14 = typedef "TSCAN_CANFD_Configuration_Regs.ctl" = cluster{"CANFD Configuration":T12, "CANFD_Sampling point":cluster{"AArbSEG1":i32, "AArbSEG2":i32, "AArbPrescaler":i32, "AArbSJW":i32, "ADataSEG1":i32, "ADataSEG2":i32, "ADataPrescaler":i32, "ADataSJW":i32}}
  T15 = typedef "Blf_Log.ctl" = cluster{"Blf_Log_PATH":path}
  T16 = typedef "UDS Cluster.ctl" = cluster{"UDS Control":T17, "DiagModuleIndex":i32}
  T17 = typedef "UDS Control.ctl" = cluster{"UDS Channel Index":u32, "Request ID":u32, "Response ID":u32, "Request ID (Func)":u32, "Session Mode":u8, "Reset Mode":u8, "DTC Mask":u8, "GropOfDTC":u32, "Seed Level":i32, "Seed":u8[], "Key Level":i32, "Key":u8[], "Read Identifier":u16, "UDS Read Data":u8[], "ASCII Data":string, "Write Identifier":u16, "UDS Wrtie Data":u8[], "IO Control Identifier":u16, "UDS IOControl Data":u8[], "IO Control Mode":u8, "UDS IOControl Read Data":u8[], "Routine Control Identifier":u16, "UDS RoutineControl Data":u8[], "UDS RoutineControl Read Data":u8[], "Routine Control Mode":u8, "SupportFDCAN":bool, "time config":cluster{"p2_timeout":i32, "p2_extended":i32, "s3_servertime":i32, "s3_clienttime":i32}, "ServiceLayer":cluster{"FilledByte":u8, "STMin":i32, "BlockSize":i32, "FCDelay":i32, "MaxLength":i32}, "Request":u8[], "Respond":u8[]}
  T18 = cluster{"MessageName":string, "SignalList":T8[]}[]
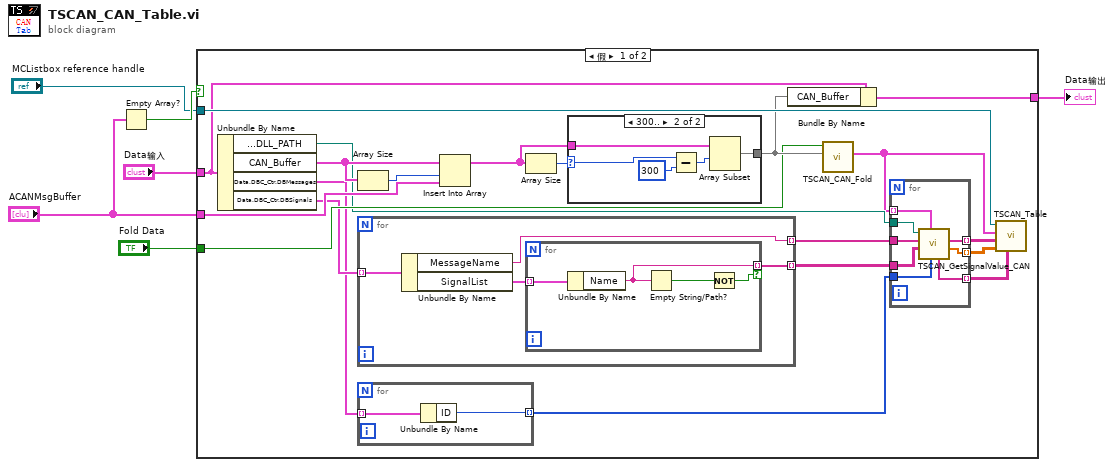
[diagram p0: block diagram]
diagram:
  n1 = Empty Array?(array="ACANMsgBuffer") -> (empty?=w4:bool)
  n2 = case shown="假" w4 {
    tunnel: "MCListbox reference handle" -> [w26 _]
    tunnel: "ACANMsgBuffer" -> [w19 _]
    tunnel: "Data输入" -> [w21 w51]
    tunnel: [w22 w51] -> w5
    tunnel: "Fold Data" -> [w17 _]
    frame False {
      n3 = Unbundle By Name(w21) -> ("Data.Config_parameter.DLL_PATH"=w14:path, "CAN_Buffer"=w20:T1, "Data.DBC_Ctr.DBMessages"=w15:T7[], "Data.DBC_Ctr.DBSignals"=w16:T18)
      n4 = Array Size(array=w20) -> (size(s)=w23:i32)
      n5 = for {
        tunnel: w16 -> [w38] mode=indexing
        tunnel: [w36] -> w13 mode=indexing
        tunnel: [w35] -> w12 mode=indexing
        n6 = Unbundle By Name(w38) -> ("MessageName"=w36:string, "SignalList"=w37:T8[])
        n7 = for {
          tunnel: w37 -> [w42] mode=indexing
          tunnel: [w41] -> w35 mode=indexing if=w39
          n8 = Unbundle By Name(w42) -> ("Name"=w41:string)
          n9 = Empty String/Path?(string/path=w41) -> (empty?=w40:bool)
          n10 = Not(x=w40) -> (.not. x?=w39:bool)
        }
      }
      n11 = for {
        tunnel: w15 -> [w44] mode=indexing
        tunnel: [w43] -> w11 mode=indexing
        n12 = Unbundle By Name(w44) -> ("ID"=w43:i32)
      }
      n13 = Insert Into Array(array=w20, index=w23, new element=w19) -> (w24:T1)
      n14 = Array Size(array=w24) -> (size(s)=w25:i32)
      n15 = case shown="300.." w25 {
        selector: w25 -> [_ w50]
        tunnel: [w45 w48] -> w18
        tunnel: w24 -> [w45 w46]
        frame 0, Default {
        }
        frame 300.. {
          n16 = Subtract(x=w50, y=300) -> (x-y=w47:i32)
          n17 = Array Subset(array=w46, index=w47) -> (w48:T1)  [unwired: 1 in]
        }
      }
      n18 = Bundle By Name(cluster=w21, "CAN_Buffer"=w18) -> (w22:T2)
      n19 = call "TSCAN_CAN_Fold.vi"("Buffer"=w18, "Fold Data"=w17) -> ("Buffer out"=w10:T1)  [unwired: 9 in]
      n20 = for {
        tunnel: w14 -> [w34]
        tunnel: w13 -> [w33]
        tunnel: w12 -> [w32]
        tunnel: w11 -> [w31]
        tunnel: w10 -> [w30] mode=indexing
        tunnel: [w29] -> w9 mode=indexing
        tunnel: [w28] -> w8 mode=indexing
        tunnel: [w27] -> w7 mode=indexing
        n21 = call "TSCAN_GetSignalValue_CAN.vi"("All_ID"=w31, "Message"=w30, "ALLSignalName"=w32, "ALLMessage"=w33, "路径输入"=w34) -> ("SigValue"=w28:dbl[], "SigName"=w29:string[], "Message Name"=w27:string[])  [unwired: 2 in, 2 out]
      }
      n22 = call "TSCAN_Table.vi"("Message Name"=w7, "SigValue"=w8, "SigName"=w9, "Buffer"=w10, "MCListbox reference handle"=w26) -> ()  [unwired: 7 in]
    }
    frame True {
    }
  }
  "Data输出" <- w5
